vi "ProdaNG.Configurator.Glb.Read.vi"(7 "DB":T2, 8 "error in (no error)":errorcluster) -> (0 "error out":errorcluster, 1 "Configuration":T1={"ShowUnreleased"=TRUE, "Param1"="StepIndex", "ParamStartIdx"=0, "Slots"=1} {"Slots" min=1 max=2; "ParamStartIdx" min=0 max=1}, 2 "Data found":bool)   [LabVIEW 2016]
uses:
  ProdaNG.Configurator.DB.ctl
  ProdaNG.Configurator.Config.ctl
  Tools/Tma.lib/nlconfig.llb/fp2ini mode.ctl
  ProdaNG.Configurator.Glb.vi
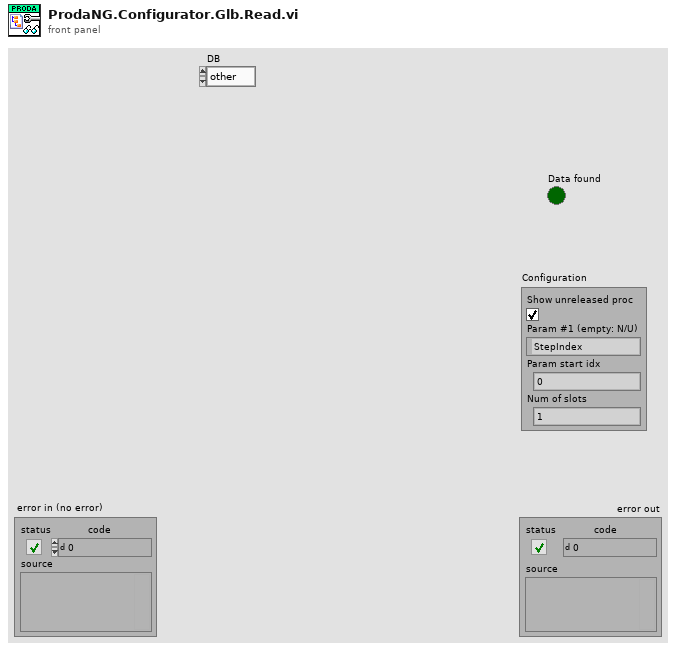
[diagram p1: front panel]
types:
  T1 = typedef "ProdaNG.Configurator.Config.ctl" = cluster{"ShowUnreleased":bool, "Param1":string, "ParamStartIdx":i32, "Slots":i32}
  T2 = typedef "ProdaNG.Configurator.DB.ctl" = enum16{"other", "WPL", "WPK"}
  T3 = typedef "fp2ini mode.ctl" = enum16{"Read Controls", "Write Controls", "Write Indicators", "Read Indicators", "Write all", "Read all"}
  T4 = enum32{"invalid app kind", "Development System", "Run Time System", "Student Edition", "Embedded LabVIEW", "Evaluation", "Custom"}
  T5 = typedef "ProdaNG.WabcoPart.ctl" = cluster{"i_id":i32, "workCenterId":i32, "contentId":string, "previewId":string, "mdReason":string, "mdUser":string, "mdTime":string, "productName":string, "wabcoNumber":string}
  T6 = typedef "ProdaNG.System.ctl" = cluster{"i_id":i32, "description":string}
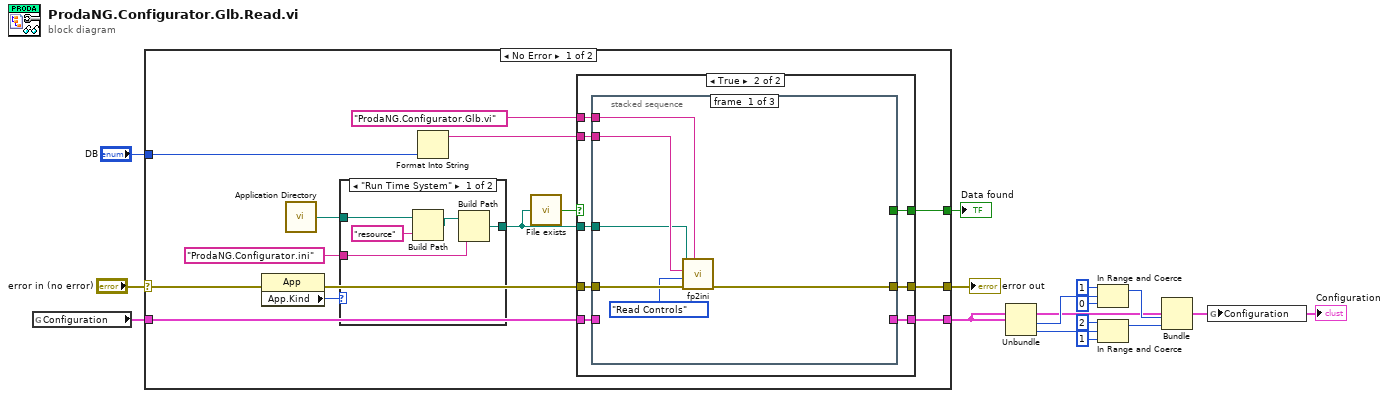
[diagram p0: block diagram]
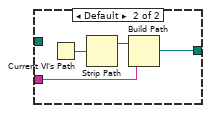
[diagram p2: hidden frame]
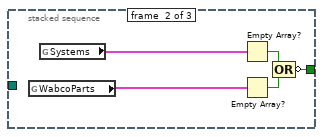
[diagram p4: hidden frame]
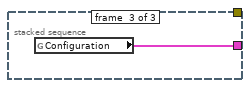
[diagram p5: hidden frame]
diagram:
  n1 = global read "ProdaNG.Configurator.Glb.vi" "Configuration"() -> (w4:T1)
  n2 = case shown="No Error" "error in (no error)" {
    selector: "error in (no error)" -> [w20 w63]
    tunnel: [w29 w63] -> w14
    tunnel: "DB" -> [w27 _]
    tunnel: [w28 _] -> w12
    tunnel: w4 -> [w22 w62]
    tunnel: [w21 w62] -> w3
    frame No Error {
      n3 = property class="App"(error in=w20) -> (error out=w19:errorcluster, "App.Kind"=w17:T4)  [unwired: 1 in, 1 out]
      n4 = call <vilib>:"Application Directory.vi"() -> ("Application Directory"=w16:path)
      n5 = case shown="\"Run Time System\"" w17 {
        tunnel: [w34 w36] -> w24
        tunnel: "ProdaNG.Configurator.ini" ("name or relative path") -> [w33 w35]
        tunnel: w16 -> [w32 _]
        frame "Run Time System" {
          n6 = Build Path(base path=w32, name or relative path="resource") -> (appended path=w31:path)
          n7 = Build Path(base path=w31, name or relative path=w33) -> (appended path=w34:path)
        }
        frame Default {
          n8 = Current VI's Path() -> (path=w38:path)
          n9 = Strip Path(path=w38) -> (stripped path=w37:path)  [unwired: 1 out]
          n10 = Build Path(base path=w37, name or relative path=w35) -> (appended path=w36:path)
        }
      }
      n11 = Format Into String(w27) -> (resulting string=w26:string)  [unwired: 3 in, 1 out]
      n12 = call "File exists.vi"("file path"=w24) -> ("exists?"=w23:bool)  [unwired: 4 in]
      n13 = case shown="True" w23 {
        selector: w23 -> [w40 _]
        tunnel: w19 -> [w41 w49]
        tunnel: [w41 w48] -> w29
        tunnel: [w40 w47] -> w28
        tunnel: w26 -> [_ w46]
        tunnel: "ProdaNG.Configurator.Glb.vi" ("name or relative path") -> [_ w45]
        tunnel: w24 -> [_ w44]
        tunnel: w22 -> [w39 w43]
        tunnel: [w39 w42] -> w21
        frame False {
        }
        frame True {
          n14 = stacked-sequence {
            tunnel: w49 -> [w55 _ _]
            tunnel: [w54 _ _] -> w48
            tunnel: [_ w56 _] -> w47
            tunnel: w46 -> [w52 _ _]
            tunnel: w45 -> [w51 _ _]
            tunnel: w44 -> [w50 _ _]
            tunnel: w43 -> [_ _ _]
            tunnel: [_ _ w61] -> w42
            frame #0 {
              n15 = call "fp2ini.vi"("vi-name (caller if empty)"=w51, "error in"=w55, "mode"=fp2ini_mode."Read Controls", "section"=w52, "ini-file path"=w50) -> ("error out"=w54:errorcluster)  [unwired: 6 in]
            }
            frame #1 {
              n16 = global read "ProdaNG.Configurator.Glb.vi" "WabcoParts"() -> (w59:T5[])
              n17 = global read "ProdaNG.Configurator.Glb.vi" "Systems"() -> (w60:T6[])
              n18 = Empty Array?(array=w60) -> (empty?=w58:bool)
              n19 = Empty Array?(array=w59) -> (empty?=w57:bool)
              n20 = Compound Arithmetic op=OR(w58, w57) -> (invert w56:bool)
            }
            frame #2 {
              n21 = global read "ProdaNG.Configurator.Glb.vi" "Configuration"() -> (w61:T1)
            }
          }
        }
      }
    }
    frame Error {
    }
  }
  "error out" <- w14
  "Data found" <- w12
  n22 = Unbundle(w3) -> ("ParamStartIdx"=w9:i32, "Slots"=w5:i32)  [unwired: 2 out]
  n23 = In Range and Coerce(upper limit=1, x=w9, lower limit=0) -> (coerced(x)=w11:i32)  [unwired: 1 out]
  n24 = In Range and Coerce(upper limit=2, x=w5, lower limit=1) -> (coerced(x)=w6:i32)  [unwired: 1 out]
  n25 = Bundle(cluster=w3, "ParamStartIdx"=w11, "Slots"=w6) -> (w2:T1)  [unwired: 2 in]
  "Configuration" <- w2
  n26 = global write "ProdaNG.Configurator.Glb.vi" "Configuration"(w2) -> ()
